vi "DPIDs.GetPIDs.vi"(8 "error in (no error)":errorcluster, 11 "Item Ref in":T1 format="%.0x") -> (0 "error out":errorcluster, 2 "PIDs":T2[](array[typedef]) {"Signals"."Byte Order" items=["Little Endian", "Big Endian"]; "Signals"."Data Type" items=["Signed", "Unsigned", "IEEE Float"]}, 3 "Section Ref out":T1 format="%.0x")   [LabVIEW 2019, in "Diagnostics Addon System Explorer.lvlib"]
uses:
  Diagnostics Addon System Explorer.lvlib
  <vilib>/NI VeriStand/Custom Device Tools/Custom Device Utility Library/Custom Device Utility Library.lvlib
  <vilib>/NI VeriStand/Custom Device Tools/Custom Device Utility Library/NI VeriStand - Search for Item by GUID.vi
  Shared/SubVIs/Constants.vi
  Shared/Diagnostics Addon Shared.lvlib
  <vilib>/NI VeriStand/Custom Device API/Custom Device API.lvlib
  Shared/Types/Signal.ctl
  Types/Frame.Export.ctl
  <vilib>/NI VeriStand/Custom Device API/Custom Device Item Ref.ctl
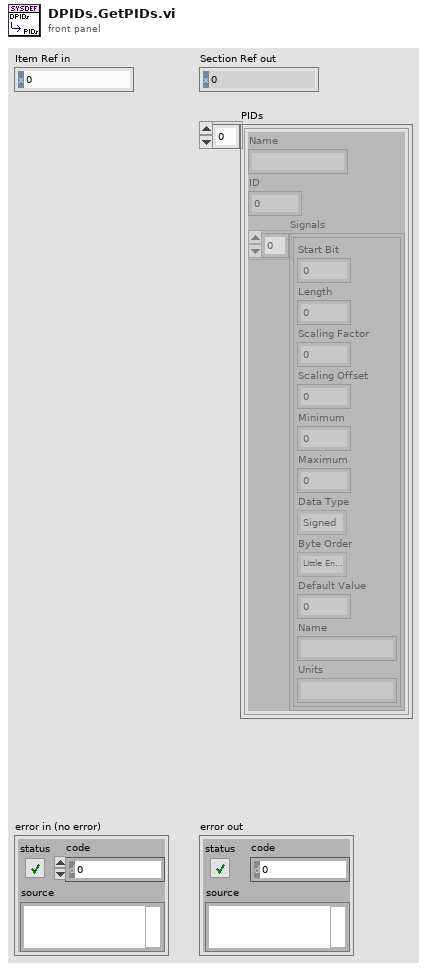
[diagram p1: front panel]
types:
  T1 = typedef "Custom Device API.lvlib/Custom Device Item Ref.ctl" = u64
  T2 = typedef "Diagnostics Addon System Explorer.lvlib/Frame.Export.ctl" = cluster{"Name":string, "ID":u32, "Signals":T3[]}
  T3 = typedef "Diagnostics Addon Shared.lvlib/Signal.ctl" = cluster{"Start Bit":u32, "Length":u32, "Scaling Factor":dbl, "Scaling Offset":dbl, "Minimum":dbl, "Maximum":dbl, "Data Type":u32, "Byte Order":u32, "Default Value":dbl, "Name":string, "Units":string}
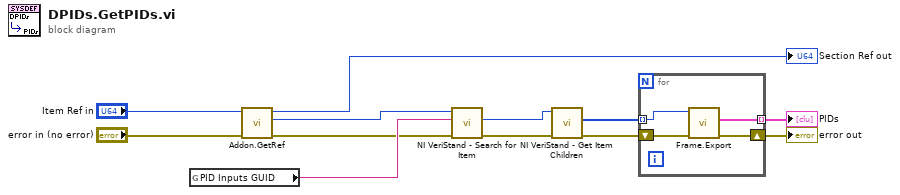
[diagram p0: block diagram]
diagram:
  n1 = global read "Constants.vi" "PID Inputs GUID"() -> (w6:string)
  n2 = call "Addon.GetRef.vi"("error in (no error)"="error in (no error)", "Node Ptr"="Item Ref in") -> ("error out"=w4:errorcluster, "Addon Ref"=w3:T1, "Node Ptr"=→"Section Ref out":T1)  [unwired: 7 in]
  n3 = call-poly <vilib>:"NI VeriStand - Search for Item.vi"("error in"=w4, "Item GUID"=w6, "Section Ref in"=w3) -> ("error out"=w7:errorcluster, "Item Ref"=w8:T1)  [unwired: 5 in, 2 out]
  n4 = call <vilib>:"NI VeriStand - Get Item Children.vi"("error in (no error)"=w7, "Item Ref in"=w8) -> ("error out"=w11:errorcluster, "Child Refs"=w10:T1[])  [unwired: 6 in, 2 out]
  n5 = for {
    tunnel: w10 -> [w16] mode=indexing
    tunnel: [w13] -> w9 mode=indexing
    shift-right: [w14] -> w12
    shift-left: w11 -> [w15]
    n6 = call "Frame.Export.vi"("error in (no error)"=w15, "Item Ref in"=w16) -> ("error out"=w14:errorcluster, "Frame"=w13:T2)  [unwired: 7 in, 1 out]
  }
  "error out" <- w12
  "PIDs" <- w9
